vi "UDP Write Byte Test.vi"() -> ()   [LabVIEW 2014, in "ESP8266 WiFi Wrapper.lvlib"]
uses:
  <vilib>/Aledyne-TSXperts/Arduino Compatible Compiler for LabVIEW/addons/ESP8266 WiFi Wrapper/ESP8266 WiFi Wrapper.lvlib
panel:
  out "Byte written?":bool
  out "Successful end packet?":bool
  out "Successful start packet?":bool
  out "Error Out":errorcluster
  in  "Error In":errorcluster
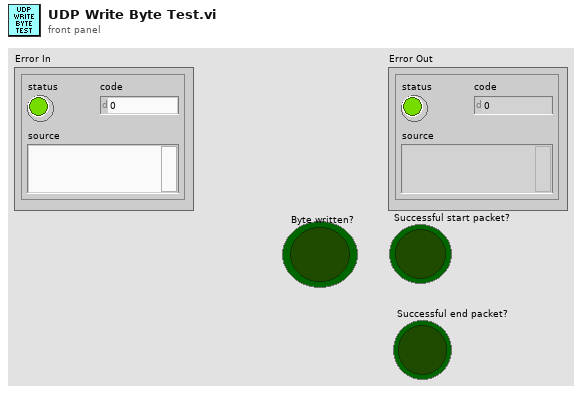
[diagram p1: front panel]
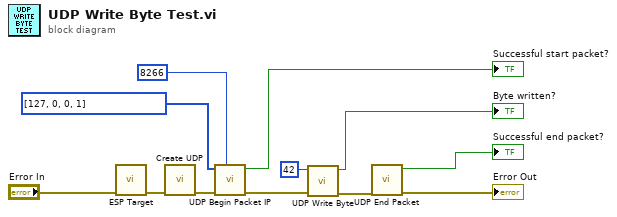
[diagram p0: block diagram]
diagram:
  n1 = call <vilib>:"ESP Target.vi"("Error In"="Error In") -> ("Error Out"=w11:errorcluster)  [unwired: 10 in]
  n2 = call <vilib>:"Create UDP.vi"("Error In"=w11) -> ("Error Out"=w10:errorcluster)  [unwired: 10 in]
  n3 = call <vilib>:"UDP Begin Packet IP.vi"("Port"=i16 8266, "Error In"=w10, "IP Address"=u8[] [127, 0, 0, 1]) -> ("Error Out"=w4:errorcluster, "Successful?"=→"Successful start packet?":bool)  [unwired: 7 in]
  n4 = call <vilib>:"UDP Write Byte.vi"("Error In"=w4, "Byte to write"=u8 42) -> ("Error Out"=w3:errorcluster, "Byte written?"=→"Byte written?":bool)  [unwired: 8 in]
  n5 = call <vilib>:"UDP End Packet.vi"("Error In"=w3) -> ("Error Out"=→"Error Out":errorcluster, "Successful?"=→"Successful end packet?":bool)  [unwired: 9 in]
